vi "emi_Splash Just display.vi"(2 "Fade/Rise time s(0)":dbl, 5 "Counter Refnum(Calling VI)":refnum<vi>, 9 "error In":errorcluster, 12 "Optional App name":string="...", 13 "Status text":string) -> (6 "Counter Refnum out":refnum<vi>, 10 "error out":errorcluster)   [LabVIEW 2011]
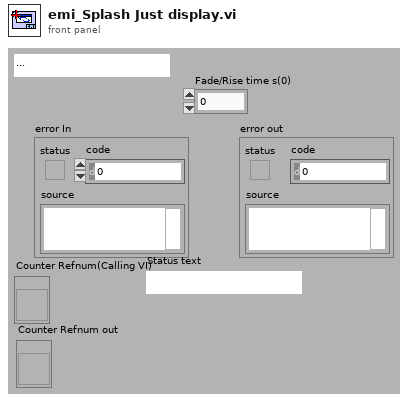
[diagram p1: front panel]
types:
  T1 = enum16{"Start", "Update", "End", "About Screen", "Just show"}
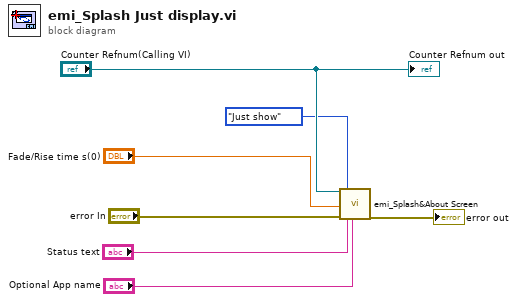
[diagram p0: block diagram]
diagram:
  n1 = call "emi_Splash&About Screen.vi"("Parrent vi during starrt(Calling VI)"="Counter Refnum(Calling VI)", "Fade/Rise time s(0)"="Fade/Rise time s(0)", "error in (no error)"="error In", "Action"=T1."Just show", "Status text"="Status text", "Optional App name"="Optional App name") -> ("error out"=→"error out":errorcluster)  [unwired: 13 in]
  "Counter Refnum out" <- "Counter Refnum(Calling VI)"
